vi "VolumeDescriptor+File.vi"(8 "error in (no error)":errorcluster) -> (0 "error out":errorcluster, 3 "VGS_VolumeDescriptor+File out":refnum<class "VGS_VolumeDescriptor+File.lvclass">)   [LabVIEW 2022 SP3, in "LV_VGS.lvlib" / "VGS_VolumeDescriptor+File.lvclass"]
uses:
  VGS_VolumeDescriptor+File.lvclass
  VGS_VolumeDescriptor+File.lvclass/VGS_VolumeDescriptor+File.ctl
  C:/Users/Andrey/Desktop/hajo/LV_VGS/vgs_project.dll
  vgs_project.dll
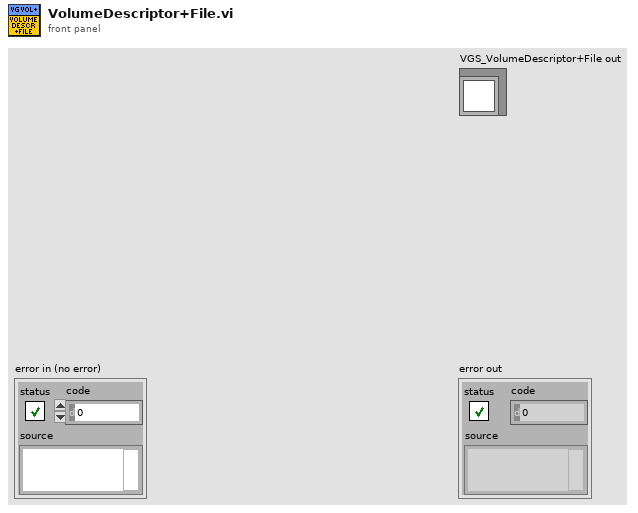
[diagram p1: front panel]
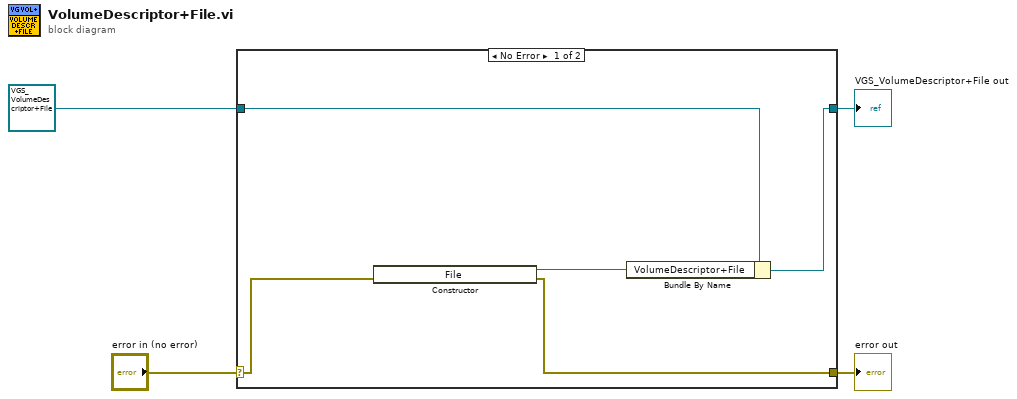
[diagram p0: block diagram]
diagram:
  n1 = case shown="No Error" "error in (no error)" {
    selector: "error in (no error)" -> [w6 w11]
    tunnel: [w5 w11] -> w3
    tunnel: [w7 w10] -> w1
    tunnel: refnum<class "VGS_VolumeDescriptor+File.lvclass"> refnum ("VGS_VolumeDescriptor+File in") -> [w9 w10]
    frame No Error {
      n2 = constructor class="VolumeDescriptor+File"(error in=w6) -> (reference out=w8:refnum<k24>, error out=w5:errorcluster)  [unwired: 2 in, 1 out]
      n3 = Bundle By Name(cluster=w9, "VolumeDescriptor+File"=w8) -> (w7:refnum<class "VGS_VolumeDescriptor+File.lvclass">)
    }
    frame Error {
    }
  }
  "error out" <- w3
  "VGS_VolumeDescriptor+File out" <- w1
